vi "OnBoard.vi"() -> ()   [LabVIEW 2020]
uses:
  <vilib>/Instr/_visa.llb/VISA Configure Serial Port (Instr).vi
panel:
  out "TYPE":string
  out "Source":string
  out "Serial Settings:Number of Bytes at Serial Port":u32
  out "Buffer From Arduino":u8[](array[numeric]) format="%x"
  in  "?":bool
  out "Sendding Buffer":u8[](array[numeric]) format="%x"
  in  "Numeric":dbl
  out "Recieced Buffer":u8[](array[numeric]) format="%x"
  out "size(s)":i32
  out "?":u8 format="%x"
  out "?":u8 format="%x"
  out "index of element":i32
  out "index of element 2":i32
  out "return count":u32
  in  "CommPort":refnum<visa-resource-name>
  out "read buffer":string
  # "OBC"
  # "Recived"
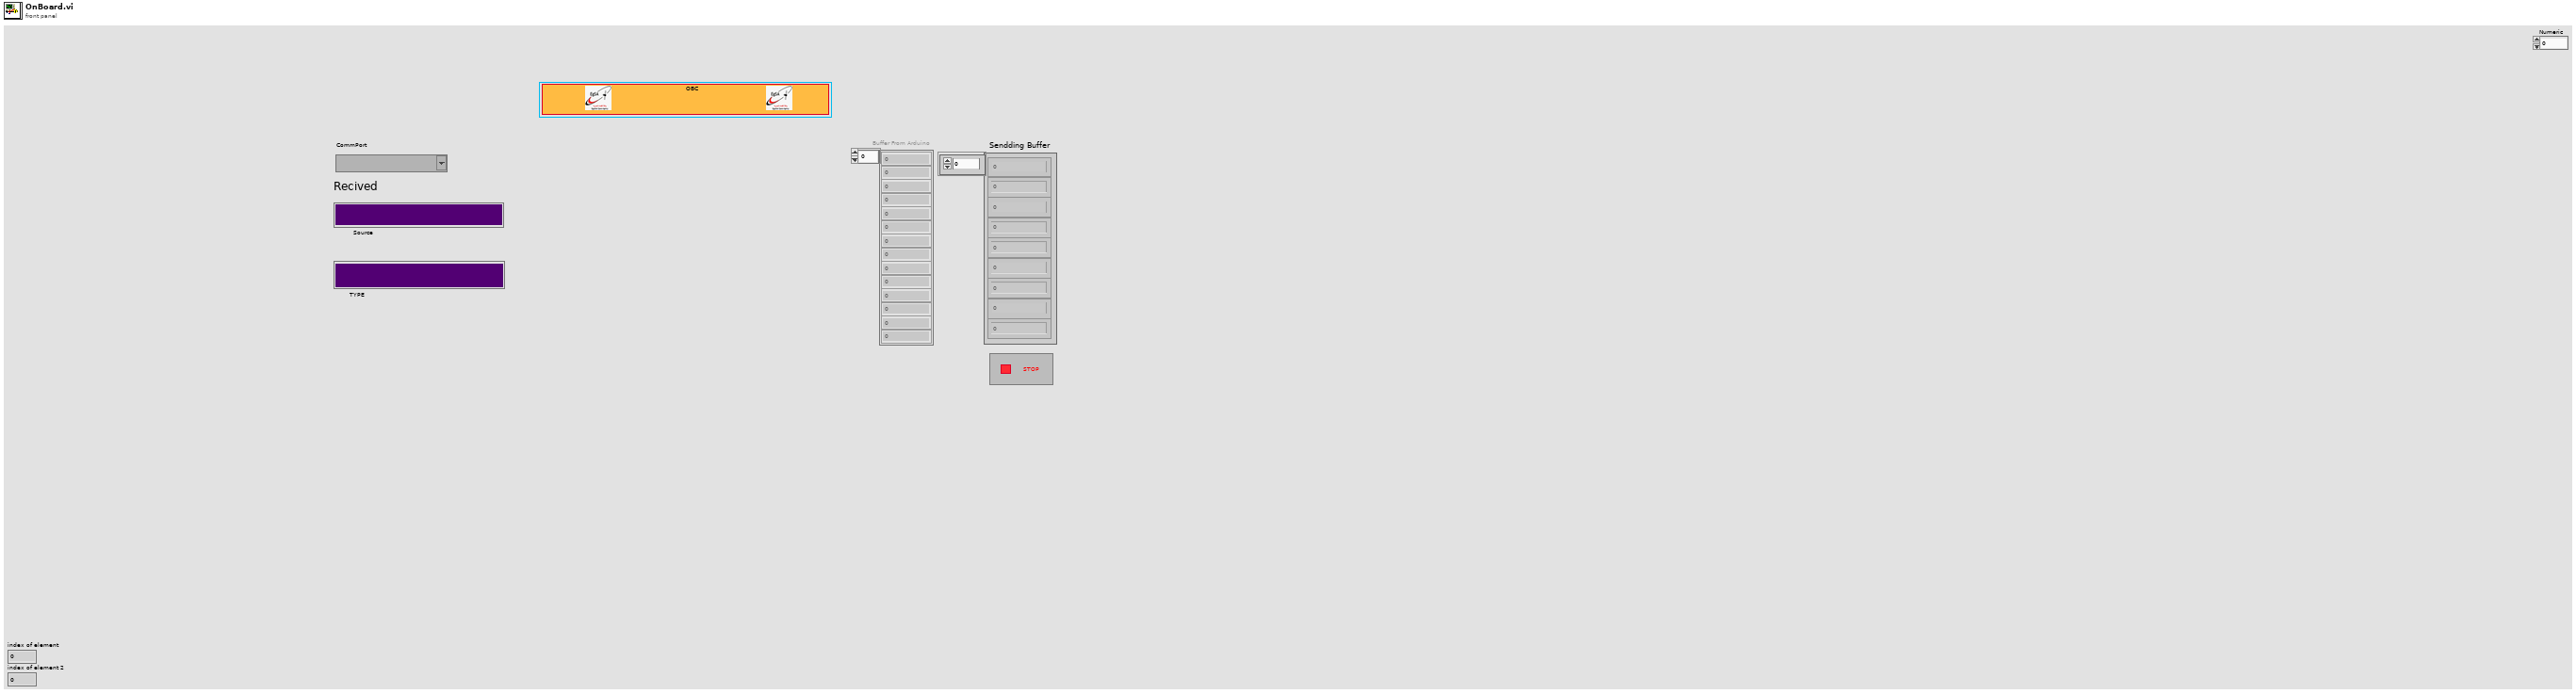
[diagram p1: front panel]
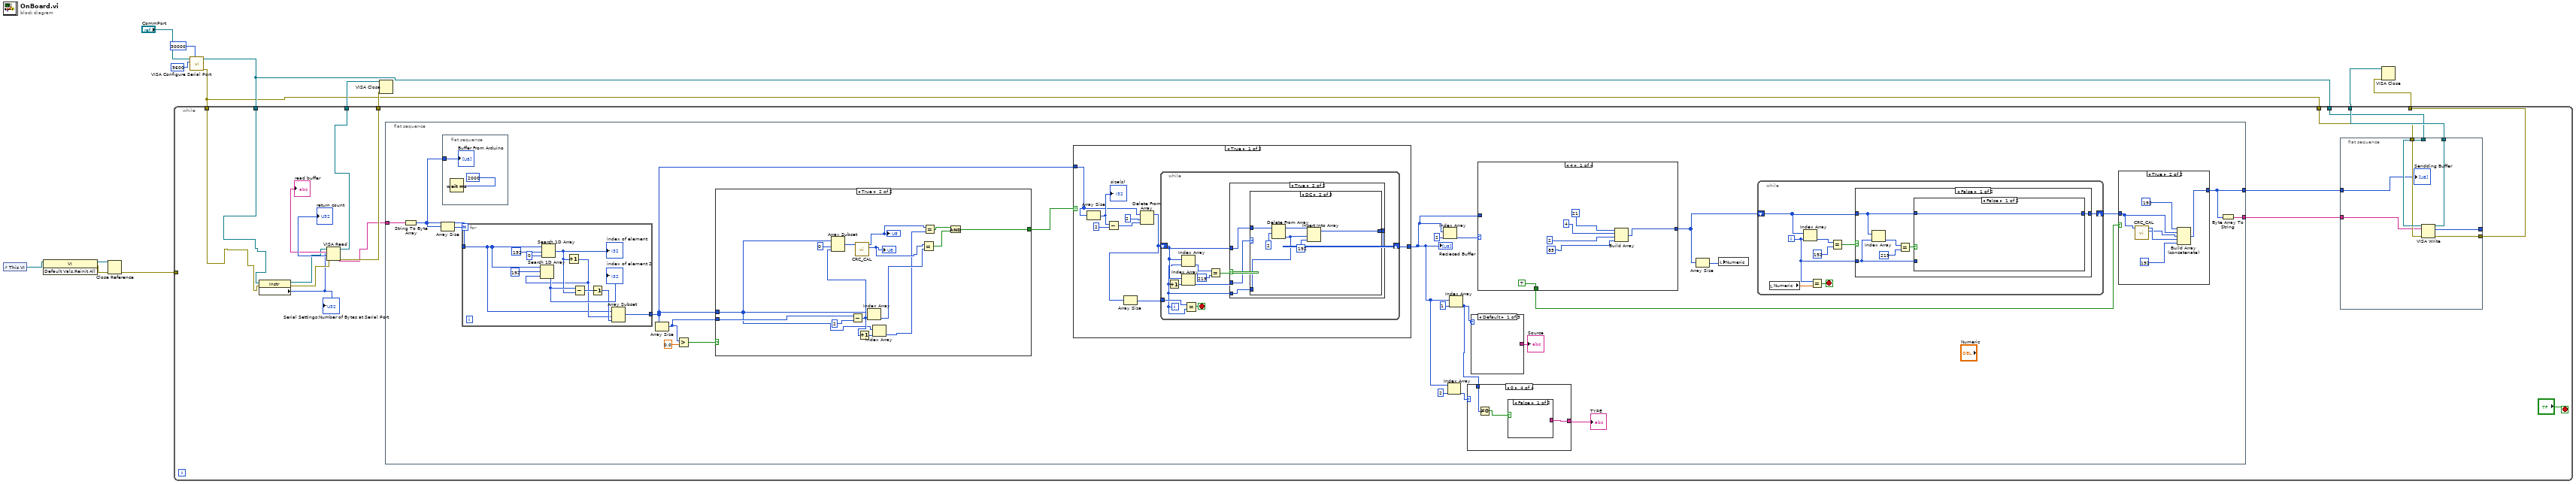
[diagram p0: block diagram]
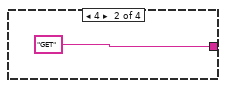
[diagram p3: hidden frame]
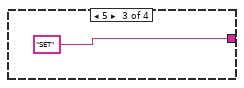
[diagram p4: hidden frame]
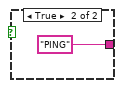
[diagram p5: hidden frame]
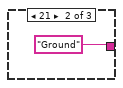
[diagram p6: hidden frame]
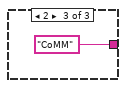
[diagram p7: hidden frame]
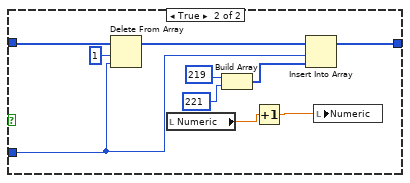
[diagram p9: hidden frame]
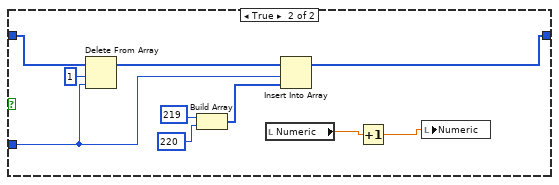
[diagram p10: hidden frame]
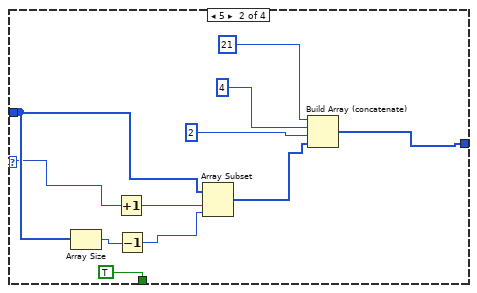
[diagram p11: hidden frame]
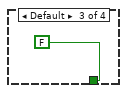
[diagram p12: hidden frame]
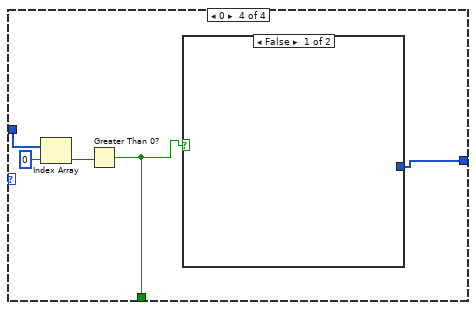
[diagram p13: hidden frame]
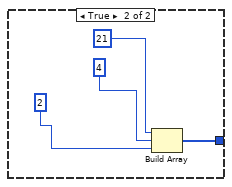
[diagram p14: hidden frame]
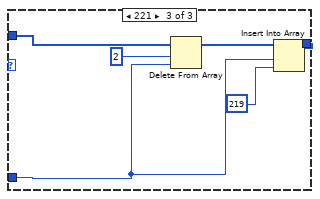
[diagram p17: hidden frame]
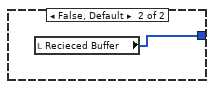
[diagram p18: hidden frame]
diagram:
  n1 = control-ref of="This VI"() -> (w2:refnum<vi>)
  n2 = invoke class="VI" method="Default Vals.Reinit All"(reference=w2) -> (reference out=w4:refnum<vi>, error out=w3:errorcluster)  [unwired: 2 in, 1 out]
  n3 = Close Reference(reference=w4, error in (no error)=w3) -> (error out=w1:errorcluster)
  n4 = call-poly "VISA Configure Serial Port"("VISA resource name"="CommPort", "timeout (10sec)"=u32 30000, "baud rate (9600)"=u32 9600) -> ("VISA resource name out"=w7:refnum<visa-resource-name>, "error out"=w6:errorcluster)  [unwired: 11 in]
  n5 = while {
    tunnel: [w28] -> w13
    tunnel: [w27] -> w12
    tunnel: w7 -> [w19]
    tunnel: w6 -> [w18]
    tunnel: [w24] -> w9
    tunnel: [w23] -> w8
    tunnel: w7 -> [w22]
    tunnel: w6 -> [w21]
    tunnel: w1 -> [_]
    stop <- "?" stop-if-true
    n6 = property class="Instr"(reference=w19, error in=w18) -> (reference out=w17:refnum<visa-resource-name>, error out=w16:errorcluster, "Serial Settings:Number of Bytes at Serial Port"=w15:u32)
    "Serial Settings:Number of Bytes at Serial Port" <- w15
    n7 = VISA Read(VISA resource name=w17, byte count=w15, error in (no error)=w16) -> (VISA resource name out=w24:refnum<visa-resource-name>, read buffer=w20:string, return count=→"return count":u32, error out=w23:errorcluster)
    "read buffer" <- w20
    n8 = flat-sequence {
      tunnel: [w38] -> w29
      tunnel: w20 -> [w46]
      tunnel: [w37] -> w14
      frame #0 {
        n9 = String To Byte Array(string=w46) -> (unsigned byte array=w47:u8[])
        n10 = Array Size(array=w47) -> (size(s)=w58:i32)
        n11 = flat-sequence {
          tunnel: w47 -> [w68]
          frame #0 {
            n12 = Wait (ms)(milliseconds to wait=u32 2000) -> ()  [unwired: 1 out]
            "Buffer From Arduino" <- w68
          }
        }
        n13 = for {
          N: w58 -> [_]
          tunnel: w47 -> [w190]
          tunnel: [w189] -> w57
          n14 = Search 1D Array(1D array=w190, element=u8 192, start index (0)=0) -> (index of element=w192:i32)
          "index of element" <- w192
          n15 = Increment(x=w192) -> (x+1=w191:i32)
          n16 = Search 1D Array(1D array=w190, element=u8 192, start index (0)=w191) -> (index of element=w195:i32)
          "index of element 2" <- w195
          n17 = Subtract(x=w195, y=w192) -> (x-y=w193:i32)
          n18 = Decrement(x=w193) -> (x-1=w194:i32)
          n19 = Array Subset(array=w190, index=w191, length=w194) -> (w189:u8[])
        }
        n20 = Array Size(array=w57) -> (size(s)=w52:i32)
        n21 = Greater?(x=w52, y=0.0) -> (0:w53:bool)
        n22 = case shown="True" w53 {
          tunnel: w52 -> [_ w188]
          tunnel: w57 -> [_ w177]
          tunnel: [_ w176] -> w56
          frame False {
          }
          frame True {
            n23 = Subtract(x=w188, y=2) -> (x-y=w182:i32)
            n24 = Array Subset(array=w177, index=0 ("length"), length=w182) -> (w183:u8[])
            n25 = call "CRC_CAL.vi"("Array"=w183) -> ("Numeric"=w180:u8, "Numeric 2"=w175:u8)  [unwired: 8 in, 1 out]
            "?" <- w180
            "?" <- w175
            n26 = Increment(x=w182) -> (x+1=w186:i32)
            n27 = Index Array(array=w177, index=w182) -> (element=w179:u8)
            n28 = Index Array(array=w177, index=w186) -> (element=w178:u8)
            n29 = Equal?(x=w180, y=w179) -> (x = y?=w185:bool)
            n30 = Equal?(x=w175, y=w178) -> (x = y?=w184:bool)
            n31 = And(x=w184, y=w185) -> (x .and. y?=w176:bool)
          }
        }
        n32 = case shown="True" w56 {
          tunnel: [w139 w174] -> w43
          tunnel: w57 -> [w138 _]
          frame True {
            n33 = Array Size(array=w138) -> (size(s)=w143:i32)
            "size(s)" <- w143
            n34 = Subtract(x=w143, y=2) -> (x-y=w144:i32)
            n35 = Delete From Array(array=w138, length=2, index=w144) -> (array with subset deleted=w145:u8[])  [unwired: 1 out]
            n36 = Array Size(array=w145) -> (size(s)=w142:i32)
            n37 = while {
              shift-right: [w147] -> w139
              shift-left: w145 -> [w148]
              tunnel: w142 -> [w155]
              i -> [w146]
              stop <- w154 stop-if-true
              n38 = Increment(x=w146) -> (x+1=w150:i32)
              n39 = Index Array(array=w148, index=w150) -> (element=w149:u8)
              n40 = Index Array(array=w148, index=w146) -> (element=w153:u8)
              n41 = Equal?(x=w155, y=w146) -> (x = y?=w154:bool)
              n42 = Equal?(x=w153, y=u8 219) -> (x = y?=w151:bool)
              n43 = case shown="True" w151 {
                tunnel: w149 -> [_ w157]
                tunnel: w148 -> [w156 w160]
                tunnel: w146 -> [_ w159]
                tunnel: [w156 w158] -> w147
                frame False {
                }
                frame True {
                  n44 = case shown="DC" w157 {
                    tunnel: w160 -> [w161 w165 w168]
                    tunnel: w159 -> [_ w163 w169]
                    tunnel: [w161 w164 w170] -> w158
                    frame Default {
                    }
                    frame 220 {
                      n45 = Delete From Array(array=w165, length=2, index=w163) -> (array with subset deleted=w166:u8[])  [unwired: 1 out]
                      n46 = Insert Into Array(array=w166, index=w163, new element=u8 192 ("y")) -> (w164:u8[])
                    }
                    frame 221 {
                      n47 = Delete From Array(array=w168, length=2, index=w169) -> (array with subset deleted=w172:u8[])  [unwired: 1 out]
                      n48 = Insert Into Array(array=w172, index=w169, new element=u8 219 ("y")) -> (w170:u8[])
                    }
                  }
                }
              }
            }
          }
          frame False, Default {
            n49 = local read "Recieced Buffer"() -> (w174:u8[])
          }
        }
        "Recieced Buffer" <- w43
        n50 = Index Array(array=w43, index=2) -> (element=w55:u8)
        n51 = Index Array(array=w43, index=2) -> (element=w40:u8)
        n52 = Index Array(array=w43, index=1) -> (element=w39:u8)
        n53 = case shown="0" w40 {
          tunnel: [_ "GET" "SET" w64] -> w41
          tunnel: w39 -> [_ _ _ w62]
          frame Default {
          }
          frame 4 {
          }
          frame 5 {
          }
          frame 0 {
            n54 = Not Equal To 0?(x=w62) -> (x != 0?=w63:bool)
            n55 = case shown="False" w63 {
              tunnel: [_ "PING"] -> w64
              frame False {
              }
              frame True {
              }
            }
          }
        }
        "TYPE" <- w41
        n56 = case shown="Default" w39 {
          tunnel: [_ "Ground" "CoMM"] -> w44
          frame Default {
          }
          frame 21 {
          }
          frame 2 {
          }
        }
        "Source" <- w44
        n57 = case shown="4" w55 {
          selector: w55 -> [_ w123 _ _]
          tunnel: w43 -> [_ w125 _ w131]
          tunnel: [w112 w118 _ w133] -> w50
          tunnel: [TRUE TRUE FALSE w129] -> w48
          frame 4 {
            n58 = Build Array(u8 21, u8 4 ("element"), u8 2, u8 85) -> (w112:u8[])
          }
          frame 5 {
            n59 = Array Size(array=w125) -> (size(s)=w126:i32)
            n60 = Increment(x=w123) -> (x+1=w124:u8)
            n61 = Decrement(x=w126) -> (x-1=w127:i32)
            n62 = Array Subset(array=w125, index=w124, length=w127) -> (w122:u8[])
            n63 = Build Array (concatenate)(u8 21, u8 4 ("element"), u8 2, w122) -> (w118:u8[])
          }
          frame Default {
          }
          frame 0 {
            n64 = Index Array(array=w131, index=0) -> (element=w130:u8)
            n65 = Greater Than 0?(x=w130) -> (x > 0?=w129:bool)
            n66 = case shown="False" w129 {
              tunnel: [_ w134] -> w133
              frame False {
              }
              frame True {
                n67 = Build Array(u8 21, u8 4 ("element"), u8 2) -> (w134:u8[])
              }
            }
          }
        }
        n68 = Array Size(array=w50) -> (size(s)=w51:i32)
        n69 = local write "Numeric"(w51) -> ()
        n70 = while {
          shift-right: [w79] -> w49
          shift-left: w50 -> [w80]
          i -> [w77]
          stop <- w78 stop-if-true
          n71 = local read "Numeric"() -> (w76:dbl)
          n72 = Index Array(array=w80, index=w77) -> (element=w83:u8)
          n73 = Equal?(x=w77, y=w76) -> (x = y?=w78:bool)
          n74 = Equal?(x=w83, y=u8 192) -> (x = y?=w81:bool)
          n75 = case shown="False" w81 {
            tunnel: w80 -> [w86 w110]
            tunnel: w77 -> [w85 w104]
            tunnel: [w84 w103] -> w79
            frame False {
              n76 = Index Array(array=w86, index=w85) -> (element=w89:u8)
              n77 = Equal?(x=w89, y=u8 219) -> (x = y?=w87:bool)
              n78 = case shown="False" w87 {
                tunnel: w86 -> [w90 w95]
                tunnel: w85 -> [_ w94]
                tunnel: [w90 w93] -> w84
                frame False {
                }
                frame True {
                  n79 = Delete From Array(array=w95, length=1, index=w94) -> (array with subset deleted=w97:u8[])  [unwired: 1 out]
                  n80 = local read "Numeric"() -> (w92:dbl)
                  n81 = Build Array(u16 219, u16 221) -> (w96:u16[])
                  n82 = Increment(x=w92) -> (x+1=w91:dbl)
                  n83 = Insert Into Array(array=w97, index=w94, new element=w96) -> (w93:u8[])
                  n84 = local write "Numeric"(w91) -> ()
                }
              }
            }
            frame True {
              n85 = Delete From Array(array=w110, length=1, index=w104) -> (array with subset deleted=w106:u8[])  [unwired: 1 out]
              n86 = Build Array(u16 219, u16 220) -> (w105:u16[])
              n87 = local read "Numeric"() -> (w101:dbl)
              n88 = Insert Into Array(array=w106, index=w104, new element=w105) -> (w103:u8[])
              n89 = Increment(x=w101) -> (x+1=w102:dbl)
              n90 = local write "Numeric"(w102) -> ()
            }
          }
        }
        n91 = case shown="True" w48 {
          tunnel: [_ w75] -> w38
          tunnel: w49 -> [_ w73]
          frame False {
          }
          frame True {
            n92 = call "CRC_CAL.vi"("Array"=w73) -> ("Numeric"=w71:u8, "Numeric 2"=w72:u8)  [unwired: 8 in, 1 out]
            n93 = Build Array (concatenate)(u8 192 ("y"), w73, w71, w72, u8 192 ("y")) -> (w75:u8[])
          }
        }
        n94 = Byte Array To String(unsigned byte array=w38) -> (string=w37:string)
      }
    }
    n95 = flat-sequence {
      tunnel: w29 -> [w30]
      tunnel: [w36] -> w28
      tunnel: [w35] -> _
      tunnel: [w34] -> w27
      tunnel: w22 -> [w33]
      tunnel: w21 -> [w32]
      tunnel: w14 -> [w31]
      frame #0 {
        n96 = VISA Write(VISA resource name=w33, write buffer=w31, error in (no error)=w32) -> (VISA resource name out=w36:refnum<visa-resource-name>, return count=w35:u32, error out=w34:errorcluster)
        "Sendding Buffer" <- w30
      }
    }
  }
  n97 = VISA Close(VISA resource name=w9, error in (no error)=w8) -> ()  [unwired: 1 out]
  n98 = VISA Close(VISA resource name=w13, error in (no error)=w12) -> ()  [unwired: 1 out]
